vi "rad_Extract Full Image.vi"(6 "Subfolder (lvappimage.contents)":string="lvappimage.contents", 8 "error in (no error)":errorcluster, 10 "App Image Temp Folder":path, 11 "Zipped App Image File Path":path) -> (0 "error out":errorcluster, 3 "Unzipped App Image Folder Path":path)   [LabVIEW 2013]
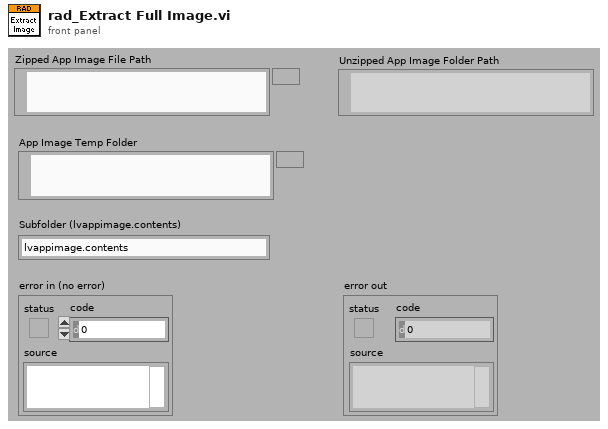
[diagram p1: front panel]
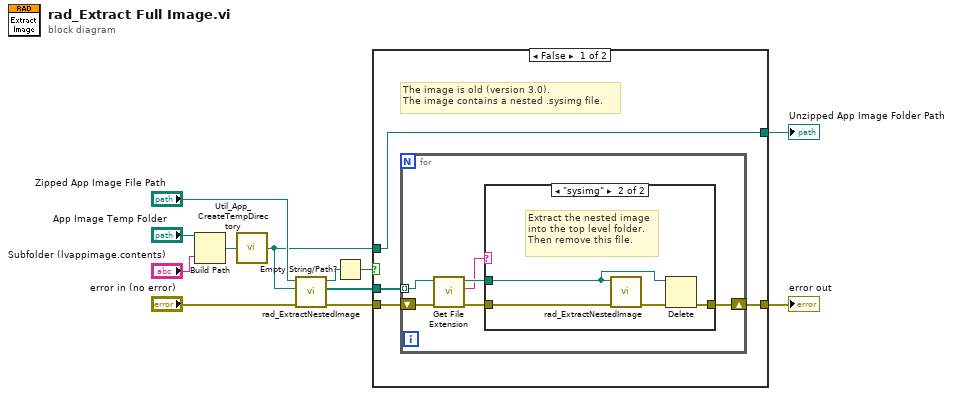
[diagram p0: block diagram]
diagram:
  n1 = Build Path(base path="App Image Temp Folder", name or relative path="Subfolder (lvappimage.contents)") -> (appended path=w11:path)
  n2 = call "Util_App_CreateTempDirectory.vi"("TempFolderPath"=w11) -> ("TempFolderPath_out"=w4:path)
  n3 = call "rad_ExtractNestedImage.vi"("error in"="error in (no error)", "TempFolderPath"=w4, "image file path"="Zipped App Image File Path") -> ("error out"=w7:errorcluster, "Unzipped files"=w5:path[], "NestedImagePath"=w9:path)  [unwired: 6 in]
  n4 = Empty String/Path?(string/path=w9) -> (empty?=w8:bool)
  n5 = case shown="False" w8 {
    tunnel: w7 -> [w15 w29]
    tunnel: [w14 w29] -> w6
    tunnel: w5 -> [w16 _]
    tunnel: w4 -> [w13 w28]
    tunnel: [w13 w28] -> w3
    frame False {
      # "The image is old (version 3.0).\nThe image contains a nested .sysimg file."
      n6 = for {
        tunnel: w16 -> [w19] mode=indexing
        shift-right: [w22] -> w14
        shift-left: w15 -> [w21]
        n7 = call <vilib>:"Get File Extension.vi"("error in (no error)"=w21, "file"=w19) -> ("error out"=w20:errorcluster, "lowercase file extension"=w17:string, "dup file"=w18:path)  [unwired: 6 in, 1 out]
        n8 = case shown="\"sysimg\"" w17 {
          tunnel: w20 -> [w23 w27]
          tunnel: w18 -> [_ w26]
          tunnel: [w23 w24] -> w22
          frame Default {
            # "Leave other files alone\nin the top level folder."
          }
          frame "sysimg" {
            # "Extract the nested image\ninto the top level folder.\nThen remove this file."
            n9 = call "rad_ExtractNestedImage.vi"("error in"=w27, "image file path"=w26) -> ("error out"=w25:errorcluster)  [unwired: 7 in, 2 out]
            n10 = Delete(path (use dialog)=w26, error in=w25) -> (error out=w24:errorcluster)  [unwired: 3 in, 2 out]
          }
        }
      }
    }
    frame True {
      # "This image is new (version 5.5).\nThe contents are compressed once."
    }
  }
  "Unzipped App Image Folder Path" <- w3
  "error out" <- w6
